vi "Access DB Path.vi"(11 "database":string="database1.mdb") -> (3 "appended path":path)   [LabVIEW 2016, in "数据查询.lvlib"]
uses:
  <vilib>/Utility/sysdir.llb/System Directory Type.ctl
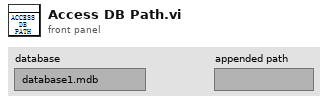
[diagram p1: front panel]
types:
  T1 = typedef "System Directory Type.ctl" = i32
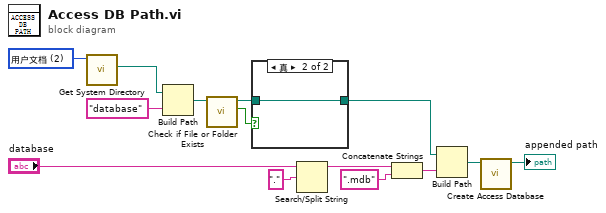
[diagram p0: block diagram]
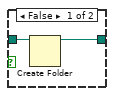
[diagram p2: hidden frame]
diagram:
  w11 = T1 2 items=["用户目录"=0, "用户桌面"=1, "用户文档"=2, "用户应用程序数据"=3, "用户设置"=4, "用户临时目录"=5, "公共文档"=6, "公共应用程序数据"=7, "公共设置"=8, "公共缓存"=13, "系统核心库"=9, "系统安装库"=10, "应用程序文件"=11, "启动盘根目录"=12] ("system directory type")
  n1 = call <vilib>:"Get System Directory.vi"("system directory type"=w11) -> ("system directory"=w10:path)  [unwired: 10 in]
  n2 = Build Path(base path=w10, name or relative path="database" ("名称或相对路径")) -> (appended path=w8:path)
  n3 = call <vilib>:"Check if File or Folder Exists.vi"("path"=w8) -> ("file or folder exists?"=w14:bool, "dup path"=w13:path)  [unwired: 8 in, 1 out]
  n4 = case shown="真" w14 {
    tunnel: w13 -> [w16 w17]
    tunnel: [w15 w17] -> w12
    frame False {
      n5 = Create Folder(path (use dialog)=w16) -> (created path=w15:path)  [unwired: 2 in, 2 out]
    }
    frame True {
    }
  }
  n6 = Search/Split String(string="database", search string/char (-)="." ("搜索字符串/字符(-)")) -> (substring before match=w3:string)  [unwired: 1 in, 2 out]
  n7 = Concatenate Strings(w3, ".mdb" ("字符串")) -> (w2:string)
  n8 = Build Path(base path=w12, name or relative path=w2) -> (appended path=w7:path)
  n9 = call "Create Access Database.vi"("路径"=w7) -> ("路径 out"=→"appended path":path)  [unwired: 9 in, 1 out]
